vi "launcher.vi"() -> ()   [LabVIEW 2020]
uses:
  modules/reporting-device/reporting-device.lvlib
panel:
  in  "show":bool
  in  "device-name":string[](array[string])=["pxi", "IC", "cRIO"]
  in  "measurements":string[][](array[string])=[["temp1", "pressure1", "distance1"], ["temp2", "pressure2", "distance2"], ["temp3", "pressure3", "distance3"], ["temp4", "", "distance4"], ["temp5", "", "distance5"], ["temp6", "", ""]]
  in  "connection":cluster{"ip":string, "port":u16, "timeout":i32}={"ip"="localhost", "port"=6379, "timeout"=1000}
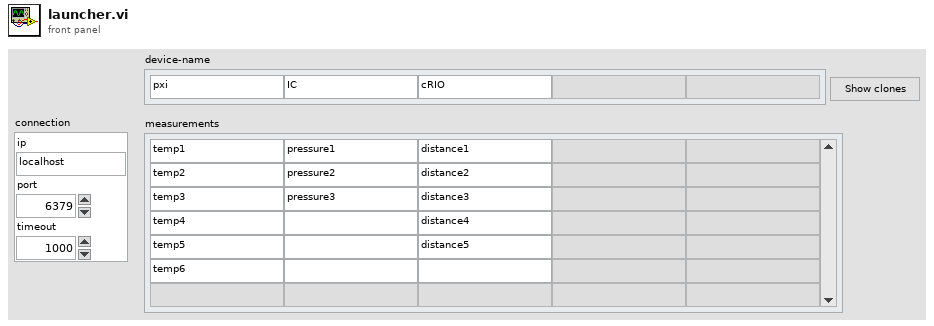
[diagram p1: front panel]
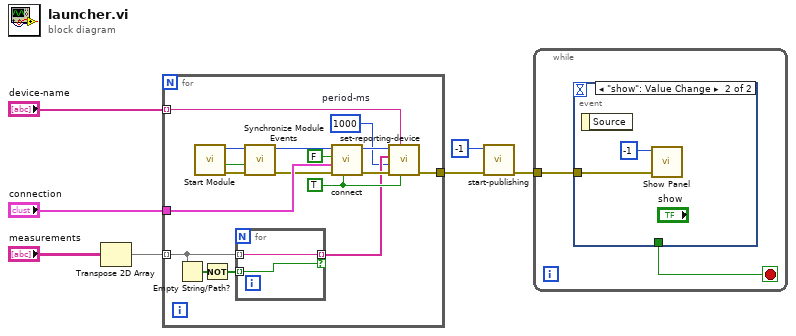
[diagram p0: block diagram]
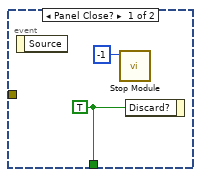
[diagram p2: hidden frame]
diagram:
  n1 = Transpose 2D Array(2D array="measurements") -> (transposed array=w5:string[][])
  n2 = for {
    tunnel: "connection" -> [w19]
    tunnel: w5 -> [w17] mode=indexing
    tunnel: [w8] -> w4
    tunnel: "device-name" -> [w9] mode=indexing
    w10 = 1000  # period-ms
    w12 = TRUE ("wait for reply (T)")
    n3 = Empty String/Path?(string/path=w17) -> (empty?=w16:bool[])
    n4 = call "Start Module.vi"() -> ("error out"=w21:errorcluster, "Wait for Event Sync?"=w22:bool, "Module ID"=w23:i32)  [unwired: 8 in, 1 out]
    n5 = Not(x=w16) -> (.not. x?=w15:bool[])
    n6 = for {
      tunnel: w17 -> [w25] mode=indexing
      tunnel: [w25] -> w11 mode=indexing if=w24
      tunnel: w15 -> [w24] mode=indexing
    }
    n7 = call "Synchronize Module Events.vi"("error in"=w21, "Wait for Event Sync?"=w22, "Module ID in"=w23) -> ("error out"=w18:errorcluster, "Module ID out"=w14:i32)  [unwired: 7 in]
    n8 = call "connect.vi"("wait for reply (T)"=w12, "error in"=w18, "connection"=w19, "flush"=FALSE, "Module ID"=w14) -> ("error out"=w13:errorcluster)  [unwired: 4 in, 2 out]
    n9 = call "set-reporting-device.vi"("wait for reply (T)"=w12, "device-name"=w9, "error in"=w13, "period-ms"=w10, "measurement-list"=w11, "Module ID"=w14) -> ("error out"=w8:errorcluster)  [unwired: 3 in, 2 out]
  }
  n10 = call "start-publishing.vi"("error in"=w4, "Module ID"=-1) -> ("error out"=w2:errorcluster)  [unwired: 6 in, 3 out]
  n11 = while {
    tunnel: w2 -> [w26]
    stop <- w27 stop-if-true
    n12 = event shown="[1] \"show\": Value Change" {
      selector: _ -> [_ _]
      dyn-events: _ -> [_ _]
      timeout: _ -> [_ _]
      tunnel: [w29 _] -> w27
      tunnel: w26 -> [_ w31]
      event Panel Close? {
        w29 = TRUE ("Discard?")
        n13 = event-data() -> ()  [unwired: 1 in, 1 out]
        n14 = call "Stop Module.vi"("Module ID"=-1) -> ()  [unwired: 10 in, 1 out]
        n15 = event-data("Discard?"=w29) -> ()  [unwired: 1 in, 1 out]
      }
      event "show": Value Change {
        n16 = event-data() -> ()  [unwired: 1 in, 1 out]
        n17 = call "Show Panel.vi"("error in"=w31, "Module ID"=-1) -> ()  [unwired: 9 in, 1 out]
      }
    }
  }
